vi "serialInit.vi"(8 "error in (no error)":errorcluster, 10 "Port":string, 11 "Python":T1) -> (0 "error out":errorcluster, 3 "Processor":enum16{"SPIKE", "Pi", "Pi_ssh"}(ring))   [LabVIEW 2019]
uses:
  Past SmartMotor UI Iterations/SerialVIs/PythonCtrl.ctl
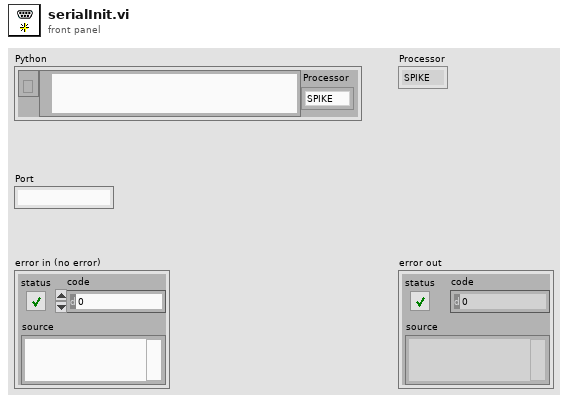
[diagram p1: front panel]
types:
  T1 = typedef "PythonCtrl.ctl" = cluster{"session":refnum<k35>, "PyPath":path, "Processor":enum16{"SPIKE", "Pi", "Pi_ssh"}}
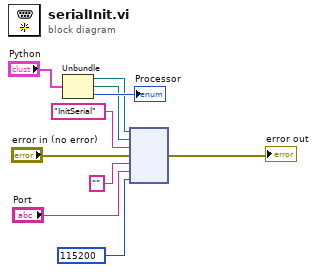
[diagram p0: block diagram]
diagram:
  n1 = Unbundle("Python") -> ("session"=w5:refnum<k35>, "PyPath"=w4:path, "Processor"=→"Processor":enum16{"SPIKE", "Pi", "Pi_ssh"})
  n2 = node(w5, w4, "InitSerial" ("function name"), "error in (no error)", "" ("function name"), "Port", 115200) -> (→"error out":errorcluster)  [unwired: 3 in, 3 out]
